vi "Evaluate File Size.vi"(8 "error in (no error)":errorcluster, 11 "Text File Sink in":refnum<class "Text File Sink.lvclass">) -> (0 "error out":errorcluster, 3 "Text File Sink out":refnum<class "Text File Sink.lvclass">)   [LabVIEW 2017, in "Text File Sink.lvclass"]
doc: "--\nCopyright © 2017 Composed SystemsI All rights reserved.\n\nAuthor: Jon McBee <jon.mcbee@composed.io>\n\nThis library is provided \"AS IS\" ,WITHOUT WARRANTIES OR\nCONDITIONS OF ANY KIND, either express or implied.\n\nComposed Systems -- composed.io\n\nStream 0.0.1.1\nJon McBee - Composed Systems\nCopyright (c) 2017, Composed Systems"
uses:
  Text File Sink.lvclass
  Text File Sink.lvclass/Text File Sink.ctl
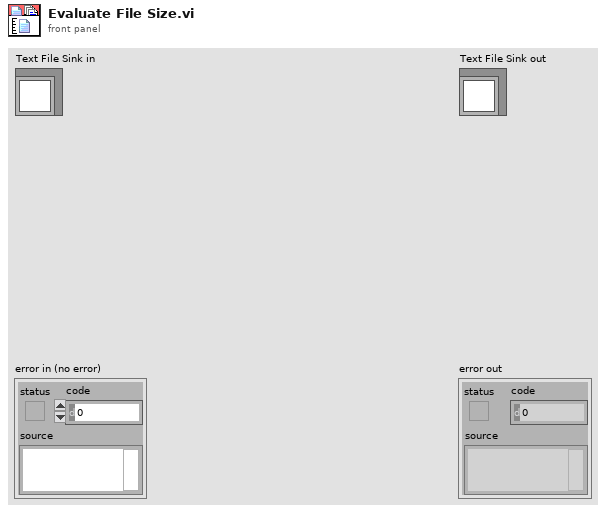
[diagram p1: front panel]
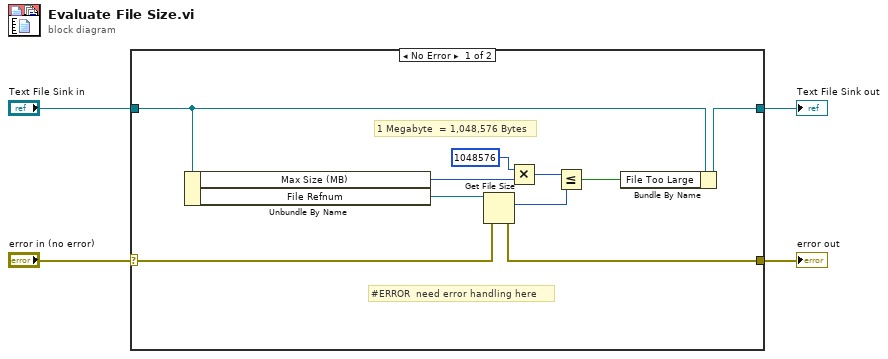
[diagram p0: block diagram]
diagram:
  n1 = case shown="No Error" "error in (no error)" {
    selector: "error in (no error)" -> [w9 w16]
    tunnel: [w8 w16] -> w3
    tunnel: [w5 w15] -> w1
    tunnel: "Text File Sink in" -> [w6 w15]
    frame No Error {
      # "#ERROR  need error handling here"
      # "1 Megabyte\t = 1,048,576 Bytes"
      n2 = Unbundle By Name(w6) -> ("Max Size (MB)"=w13:i64, "File Refnum"=w14:refnum<file>)
      n3 = Get File Size(file=w14, error in=w9) -> (size (in bytes)=w10:i64, 0:w8:errorcluster)  [unwired: 1 out]
      n4 = Multiply(x=i64 1048576 ("y"), y=w13) -> (x*y=w11:i64)
      n5 = Less Or Equal?(x=w11, y=w10) -> (x <= y?=w7:bool)
      n6 = Bundle By Name(cluster=w6, "File Too Large"=w7) -> (w5:refnum<class "Text File Sink.lvclass">)
    }
    frame Error {
    }
  }
  "error out" <- w3
  "Text File Sink out" <- w1
